vi "读小信号变比.vi"(11 "串口号":refnum<visa-resource-name>) -> (10 "应答":string)   [LabVIEW 2014]
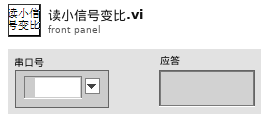
[diagram p1: front panel]
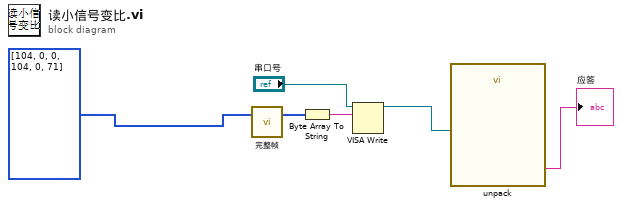
[diagram p0: block diagram]
diagram:
  n1 = call "完整帧.vi"("不完整帧"=u8[] [104, 0, 0, 104, 0, 71]) -> ("完整帧"=w6:u8[])  [unwired: 2 in]
  n2 = Byte Array To String(unsigned byte array=w6) -> (string=w5:string)
  n3 = VISA Write(VISA resource name="串口号", write buffer=w5) -> (VISA resource name out=w3:refnum<visa-resource-name>)  [unwired: 1 in, 2 out]
  n4 = call "unpack.vi"("串口号输入"=w3) -> ("应答"=→"应答":string)  [unwired: 5 in, 1 out]
